vi "LVCAM Write Self Actor.vi"(10 "Self Actor":refnum<class "LVCAM.lvclass">, 11 "Self Actor in":refnum<class "Self Actor.lvclass">) -> (3 "Self Actor out":refnum<class "Self Actor.lvclass">)   [LabVIEW 2021, in "LVCAM.lvlib" / "Self Actor.lvclass"]
uses:
  Self Actor.lvclass
  LVCAM/LVCAM.lvclass
  Msgs/LVCAM Destroy Self/LVCAM Destroy Self Msg/LVCAM Destroy Self Msg.lvclass
  Self Msg Send.vi
  C:/PPLs/LabVIEW-Composed-Actor-Model-LVCAM/LabVIEW-Composed-Actor-Model-LVCAM/LVCAM/LVCAM/LVCAM/LVCAM.lvclass
  C:/PPLs/LabVIEW-Composed-Actor-Model-LVCAM/LabVIEW-Composed-Actor-Model-LVCAM/LVCAM/Msgs/LVCAM Create Nest/LVCAM Create Nest/LVCAM Create Nest.lvclass
  C:/PPLs/LabVIEW-Composed-Actor-Model-LVCAM/LabVIEW-Composed-Actor-Model-LVCAM/LVCAM/Msgs/LVCAM Destroy Self/LVCAM Destroy Self/LVCAM Destroy Self.lvclass
  C:/PPLs/LabVIEW-Composed-Actor-Model-LVCAM/LabVIEW-Composed-Actor-Model-LVCAM/LVCAM/Msgs/LVCAM Nest Destroyed/LVCAM Nest Destroyed/LVCAM Nest Destroyed.lvclass
  C:/PPLs/LabVIEW-Composed-Actor-Model-LVCAM/LabVIEW-Composed-Actor-Model-LVCAM/LVCAM/LVCAM/LVCAM Msg Drop/LVCAM Msg Drop.lvclass
  C:/PPLs/LabVIEW-Composed-Actor-Model-LVCAM/LabVIEW-Composed-Actor-Model-LVCAM/LVCAM/LVCAM/LVCAM Msg Receive/LVCAM Msg Receive.lvclass
  C:/PPLs/LabVIEW-Composed-Actor-Model-LVCAM/LabVIEW-Composed-Actor-Model-LVCAM/LVCAM/LVCAM/LVCAM Propagate Error/LVCAM Propagate Error.lvclass
  C:/PPLs/LabVIEW-Composed-Actor-Model-LVCAM/LabVIEW-Composed-Actor-Model-LVCAM/LVCAM/LVCAM/LVCAM Write Self Actor/LVCAM Write Self Actor.lvclass
  C:/PPLs/LabVIEW-Composed-Actor-Model-LVCAM/LabVIEW-Composed-Actor-Model-LVCAM/LVCAM/LVCAM/Self Actor/Self Actor.lvclass
  C:/PPLs/LabVIEW-Composed-Actor-Model-LVCAM/LabVIEW-Composed-Actor-Model-LVCAM/LVCAM/LVCAM/Msg Q/Msg Q.lvclass
  C:/PPLs/LabVIEW-Composed-Actor-Model-LVCAM/LabVIEW-Composed-Actor-Model-LVCAM/LVCAM/Msgs/LVCAM Destroy Self/LVCAM Destroy Self Msg/LVCAM Destroy Self Msg.lvclass
  C:/PPLs/LabVIEW-Composed-Actor-Model-LVCAM/LabVIEW-Composed-Actor-Model-LVCAM/LVCAM/LVCAM/Msg/Msg.lvclass
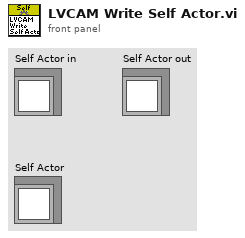
[diagram p1: front panel]
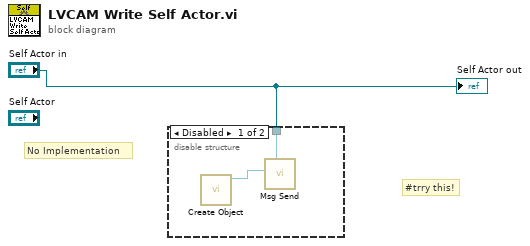
[diagram p0: block diagram]
diagram:
  # "#trry this!"
  # "No Implementation"
  n1 = disable-structure shown="Disabled" {
    disable-tunnel: "Self Actor in" -> [w3 _]
    frame Disabled {
      n2 = call "Create Object.vi"() -> ("LVCAM Destroy Self Msg out"=w2:refnum<class "LVCAM Destroy Self Msg.lvclass">)  [unwired: 11 in]
      n3 = call-poly "Msg Send.vi"("Self Actor"=w3, "Msg"=w2) -> ()  [unwired: 9 in, 1 out]
    }
    frame Enabled {
    }
  }
  "Self Actor out" <- "Self Actor in"
